vi "Clapper.vi"(7 "State":T4=enum."Out", 8 "Error in":errorcluster, 10 "Plugged":T1={"DevStatus"={"status"=FALSE, "code"=0, "source"=""}, "Solenoid Module"=enum."Solenoid Module 1", "Forward Solenoid Channel"=enum."Invalid", "Reverse Solenoid Channel"=enum."Invalid"}, 11 "Open":T1={"DevStatus"={"status"=FALSE, "code"=0, "source"=""}, "Solenoid Module"=enum."Solenoid Module 1", "Forward Solenoid Channel"=enum."Invalid", "Reverse Solenoid Channel"=enum."Invalid"}) -> (0 "Error out":errorcluster)   [LabVIEW 2013]
doc: "VI for the clapper double solenoid. It has the following actions:\n-Init: take a reference to a double solenoid and store it in a shift register so that it does not need to be passed in again.\n-In: sets the cylinder to the in position.\n-Middle: set the cylinder to the middle position.\n-Out: set the cylinder to the out position."
uses:
  <vilib>/Rock Robotics/WPI/Solenoid/WPI_SolenoidDevRef.ctl
  <vilib>/Rock Robotics/SystemInterfaces/Typedef/FPGA_TypedefSolenoidModule.ctl
  <vilib>/Rock Robotics/WPI/Solenoid/WPI_SolenoidChannel.ctl
  DoubleSolenoidAction.ctl
  <vilib>/Rock Robotics/WPI/Solenoid/WPI_SolenoidValue.ctl
  <vilib>/Rock Robotics/WPI/Solenoid/WPI_SolenoidSetEnum.vi
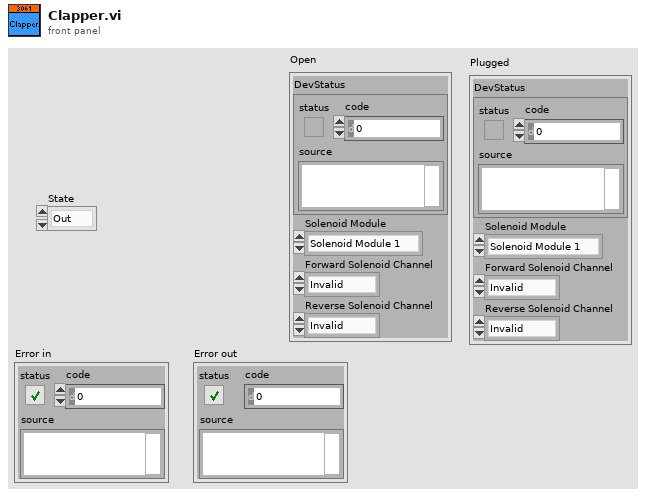
[diagram p1: front panel]
types:
  T1 = typedef "WPI_SolenoidDevRef.ctl" = cluster{"DevStatus":errorcluster, "Solenoid Module":T2, "Forward Solenoid Channel":T3, "Reverse Solenoid Channel":T3}
  T2 = typedef "FPGA_TypedefSolenoidModule.ctl" = enum16{"Solenoid Module 1", "Solenoid Module 2"}
  T3 = typedef "WPI_SolenoidChannel.ctl" = enum8{"Solenoid 1", "Solenoid 2", "Solenoid 3", "Solenoid 4", "Solenoid 5", "Solenoid 6", "Solenoid 7", "Solenoid 8", "Invalid"}
  T4 = typedef "DoubleSolenoidAction.ctl" = enum16{"Init", "Middle", "In", "Out"}
  T5 = typedef "WPI_SolenoidValue.ctl" = enum16{"Off", "On", "Forward", "Reverse"}
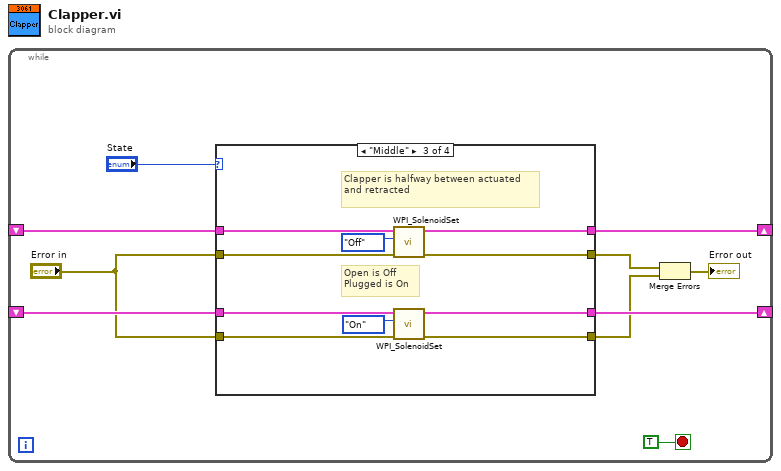
[diagram p0: block diagram]
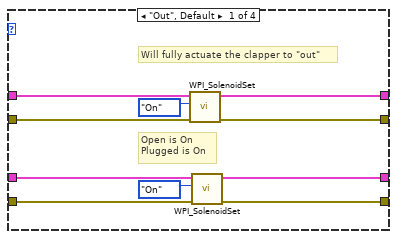
[diagram p2: hidden frame]
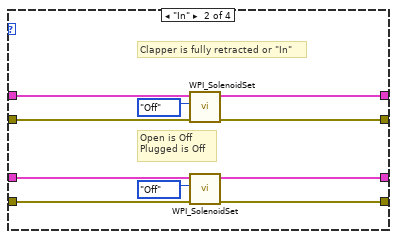
[diagram p3: hidden frame]
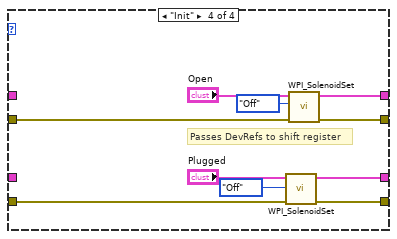
[diagram p4: hidden frame]
diagram:
  n1 = while {
    shift-right: [w8] -> _
    shift-left: _ -> [w7]
    shift-right: [w5] -> _
    shift-left: _ -> [w4]
    stop <- TRUE stop-if-true
    n2 = case shown="\"Middle\"" "State" {
      tunnel: [w20 w30 w40 w49] -> w8
      tunnel: w7 -> [w18 w28 w39 _]
      tunnel: "Error in" -> [w17 w27 w38 w47]
      tunnel: [w16 w26 w37 w46] -> w6
      tunnel: [w14 w24 w34 w44] -> w5
      tunnel: w4 -> [w15 w25 w35 _]
      tunnel: "Error in" -> [w12 w23 w32 w43]
      tunnel: [w11 w22 w33 w42] -> w1
      frame "Out", Default {
        # "Open is On\nPlugged is On"
        # "Will fully actuate the clapper to \"out\""
        n3 = call-poly <vilib>:"WPI_SolenoidSet.vi"("error in (no error)"=w17, "Value"=WPI_SolenoidValue."On", "SolenoidDevRef"=w18) -> ("error out"=w16:errorcluster, "SolenoidDevRef"=w20:T1)  [unwired: 7 in]
        n4 = call-poly <vilib>:"WPI_SolenoidSet.vi"("error in (no error)"=w12, "Value"=WPI_SolenoidValue."On", "SolenoidDevRef"=w15) -> ("error out"=w11:errorcluster, "SolenoidDevRef"=w14:T1)  [unwired: 7 in]
      }
      frame "In" {
        # "Open is Off\nPlugged is Off"
        # "Clapper is fully retracted or \"In\""
        n5 = call-poly <vilib>:"WPI_SolenoidSet.vi"("error in (no error)"=w27, "Value"=WPI_SolenoidValue."Off", "SolenoidDevRef"=w28) -> ("error out"=w26:errorcluster, "SolenoidDevRef"=w30:T1)  [unwired: 7 in]
        n6 = call-poly <vilib>:"WPI_SolenoidSet.vi"("error in (no error)"=w23, "Value"=WPI_SolenoidValue."Off", "SolenoidDevRef"=w25) -> ("error out"=w22:errorcluster, "SolenoidDevRef"=w24:T1)  [unwired: 7 in]
      }
      frame "Middle" {
        # "Open is Off\nPlugged is On"
        # "Clapper is halfway between actuated and retracted"
        n7 = call-poly <vilib>:"WPI_SolenoidSet.vi"("error in (no error)"=w38, "Value"=WPI_SolenoidValue."Off", "SolenoidDevRef"=w39) -> ("error out"=w37:errorcluster, "SolenoidDevRef"=w40:T1)  [unwired: 7 in]
        n8 = call-poly <vilib>:"WPI_SolenoidSet.vi"("error in (no error)"=w32, "Value"=WPI_SolenoidValue."On", "SolenoidDevRef"=w35) -> ("error out"=w33:errorcluster, "SolenoidDevRef"=w34:T1)  [unwired: 7 in]
      }
      frame "Init" {
        # "Passes DevRefs to shift register"
        n9 = call-poly <vilib>:"WPI_SolenoidSet.vi"("error in (no error)"=w43, "Value"=WPI_SolenoidValue."Off", "SolenoidDevRef"="Plugged") -> ("error out"=w42:errorcluster, "SolenoidDevRef"=w44:T1)  [unwired: 7 in]
        n10 = call-poly <vilib>:"WPI_SolenoidSet.vi"("error in (no error)"=w47, "Value"=WPI_SolenoidValue."Off", "SolenoidDevRef"="Open") -> ("error out"=w46:errorcluster, "SolenoidDevRef"=w49:T1)  [unwired: 7 in]
      }
    }
    n11 = Merge Errors(w6, w1) -> (→"Error out":errorcluster)
  }
